vi "test BroadcastRegistry.vi"() -> ()   [LabVIEW 2017]
uses:
  user.lib/_NEVSTOP/Communicable State Machine(CSM)/_Support/FGV-BroadcastRegistry/Operation-BroadcastRegistry.ctl
  user.lib/_NEVSTOP/Communicable State Machine(CSM)/Communicable State Machine.lvlib
panel:
  out "response message":string[](array[string])
  out "response message":string[](array[string])
  out "response message":string[](array[string])
  out "response message":string[](array[string])
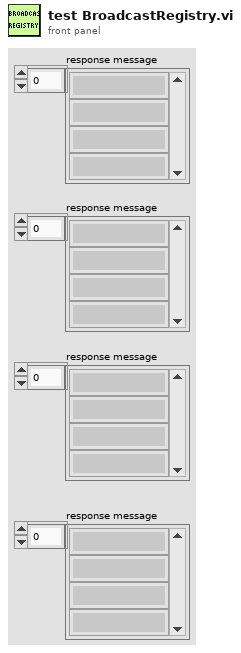
[diagram p1: front panel]
types:
  T1 = typedef "Communicable State Machine.lvlib/Operation-BroadcastRegistry.ctl" = enum16{"Delete Source Module", "Delete Target Module", "Remove Module", "Register", "Unregister", "Check"}
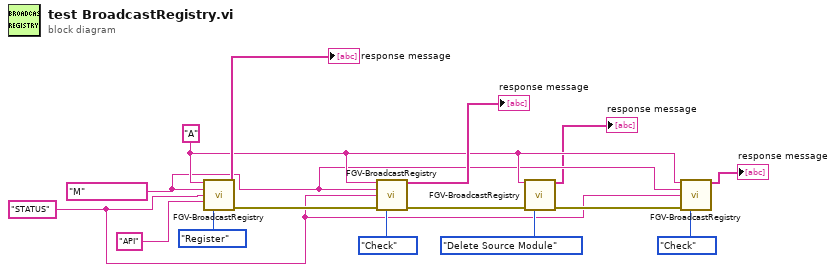
[diagram p0: block diagram]
diagram:
  w3 = "STATUS" ("Message")
  w4 = "M" ("Dest")
  w5 = "A" ("Source")
  n1 = call "FGV-BroadcastRegistry.vi"("Source"=w5, "Target"=w4, "Status"=w3, "API"="API" ("Response Message In"), "Operation"=Operation-BroadcastRegistry."Register") -> ("response message"=→"response message":string[], "Error out"=w12:errorcluster)  [unwired: 9 in]
  n2 = call "FGV-BroadcastRegistry.vi"("Source"=w5, "Target"=w4, "Status"=w3, "Error in"=w12, "Operation"=Operation-BroadcastRegistry."Check") -> ("response message"=→"response message":string[], "Error out"=w9:errorcluster)  [unwired: 9 in]
  n3 = call "FGV-BroadcastRegistry.vi"("Source"=w5, "Error in"=w9, "Operation"=Operation-BroadcastRegistry."Delete Source Module") -> ("response message"=→"response message":string[], "Error out"=w6:errorcluster)  [unwired: 11 in]
  n4 = call "FGV-BroadcastRegistry.vi"("Source"=w5, "Target"=w4, "Status"=w3, "Error in"=w6, "Operation"=Operation-BroadcastRegistry."Check") -> ("response message"=→"response message":string[])  [unwired: 9 in, 1 out]
